vi "Bearbeiter_triggern.vi"(10 "automatisch out":T1, 11 "Bearbeiter (Eingang)":refnum<vi>) -> ()   [LabVIEW 2020, in "Linearisierung v2.lvlib" / "SpanEinstellungen.lvlib"]
uses:
  SpanEinstellungen.lvlib
  Seiten/System Einstellungen V2/Konfig Gasflasche.ctl
  Seiten/System Einstellungen V2/System Einstellungen V2.lvlib
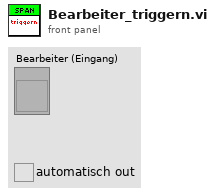
[diagram p1: front panel]
types:
  T1 = typedef "System Einstellungen V2.lvlib/Konfig Gasflasche.ctl" = bool
  T2 = typedef "String - Eingabefeld.ctl" = string
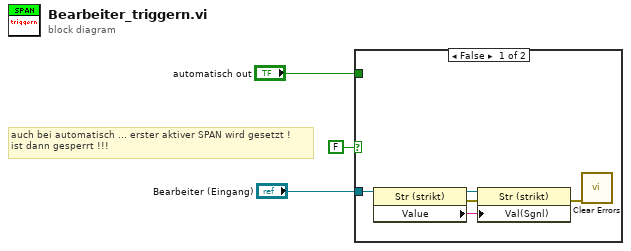
[diagram p0: block diagram]
diagram:
  # "auch bei automatisch ... erster aktiver SPAN wird gesetzt !\nist dann gesperrt !!!"
  n1 = case shown="False" FALSE {
    tunnel: "automatisch out" -> [_ _]
    tunnel: "Bearbeiter (Eingang)" -> [w8 _]
    frame False {
      n2 = property class="Str (strikt)"(reference=w8) -> (reference out=w7:refnum<vi>, error out=w6:errorcluster, "Value"=w4:T2)  [unwired: 1 in]
      n3 = property class="Str (strikt)"(reference=w7, error in=w6, "Val(Sgnl)"=w4) -> (error out=w5:errorcluster)  [unwired: 1 out]
      n4 = call <vilib>:"Clear Errors.vi"("error in (no error)"=w5) -> ()  [unwired: 5 in, 2 out]
    }
    frame True {
    }
  }
